vi "Pre Launch Init.vi"(11 "GlobalPlannerPyPl in":refnum<class "GlobalPlannerPyPl.lvclass"> caption="操作者输入") -> (0 "error out":errorcluster caption="错误输出", 3 "GlobalPlannerPyPl out":refnum<class "GlobalPlannerPyPl.lvclass"> caption="操作者输出")   [LabVIEW 2014, in "GlobalPlannerPyPl.lvlib" / "GlobalPlannerPyPl.lvclass"]
doc: "(<B>Filename</B>: Actor Framework.lvlib:Actor.lvclass:Pre Launch Init.vi)\n\nDefines behavior that occurs after the Launch Nested Actor method is invoked but before the actor's Actor Core method begins running.\n\nBy default, this method does nothing. A descendant class may override it to define behavior."
uses:
  GlobalPlannerPyPl.lvclass
  Global_var/Global_var.vi
  Wrapper_lib/zsActor/ActorWrapper.lvclass
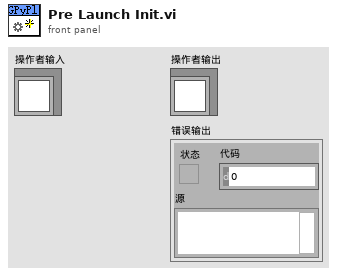
[diagram p1: front panel]
types:
  T1 = typedef "Point.ctl" = cluster{"x":dbl, "y":dbl, "z":dbl}
  T2 = typedef "P3AT_Current.ctl" = cluster{"max_vel":dbl, "max_rot":dbl, "now_pose_X":dbl, "now_pose_Y":dbl, "now_pose_Rot_deg":dbl, "Control_Mode":enum32{"Joy", "Map", "Voice", "Input", "Undefined"}}
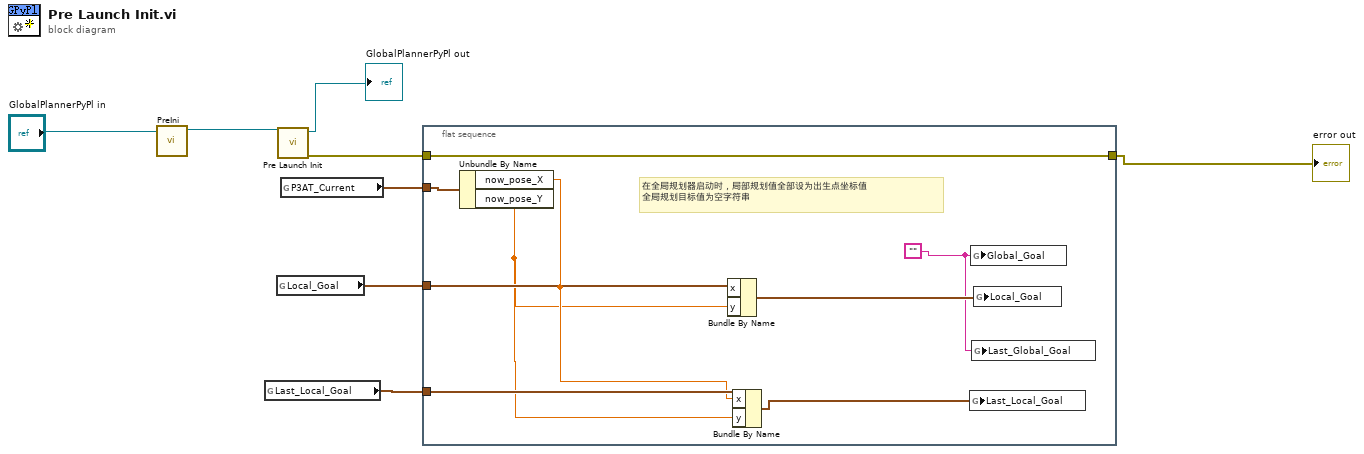
[diagram p0: block diagram]
diagram:
  n1 = call "PreIni.vi"("zsActor输入"="GlobalPlannerPyPl in") -> ("zsActor输出"=w4:refnum<class "GlobalPlannerPyPl.lvclass">)  [unwired: 9 in, 1 out]
  n2 = global read "Global_var.vi" "Last_Local_Goal"() -> (w5:T1)
  n3 = global read "Global_var.vi" "Local_Goal"() -> (w6:T1)
  n4 = call-parent "Pre Launch Init.vi"("Actor in"=w4) -> ("error out"=w8:errorcluster, "Actor out"=→"GlobalPlannerPyPl out":refnum<class "GlobalPlannerPyPl.lvclass">)  [unwired: 9 in]
  n5 = global read "Global_var.vi" "P3AT_Current"() -> (w7:T2)
  n6 = flat-sequence {
    tunnel: w8 -> [w17]
    tunnel: [w17] -> w1
    tunnel: w7 -> [w16]
    tunnel: w6 -> [w15]
    tunnel: w5 -> [w14]
    frame #0 {
      w9 = ""
      # "在全局规划器启动时，局部规划值全部设为出生点坐标值\n全局规划目标值为空字符串"
      n7 = Unbundle By Name(w16) -> ("now_pose_X"=w13:dbl, "now_pose_Y"=w12:dbl)
      n8 = Bundle By Name(cluster=w15, "x"=w13, "y"=w12) -> (w11:T1)
      n9 = Bundle By Name(cluster=w14, "x"=w13, "y"=w12) -> (w10:T1)
      n10 = global write "Global_var.vi" "Last_Local_Goal"(w10) -> ()
      n11 = global write "Global_var.vi" "Global_Goal"(w9) -> ()
      n12 = global write "Global_var.vi" "Last_Global_Goal"(w9) -> ()
      n13 = global write "Global_var.vi" "Local_Goal"(w11) -> ()
    }
  }
  "error out" <- w1
